vi "senix sonic.vi"() -> ()   [LabVIEW 2014]
uses:
  <vilib>/Instr/_visa.llb/VISA Flush IO Buffer Mask.ctl
  <vilib>/Instr/_visa.llb/VISA Configure Serial Port (Instr).vi
panel:
  out "Waveform Chart":dbl(graph)
  out "Distance, in":dbl
  in  "stop":bool
  out "error out":errorcluster
  out "return count":u32
  out "read buffer":string
  in  "VISA resource name":refnum<visa-resource-name>="COM3"
  # "This vi reads a continuous stream of data from the Senix Sonix sensor TSPC-30S1-232\nThe sensor has been configured to stream continuous data using their software SenixView.\nThe serial port setup values are the default for the Senix sensor."
  # "The value 0000 represent \"no read\""
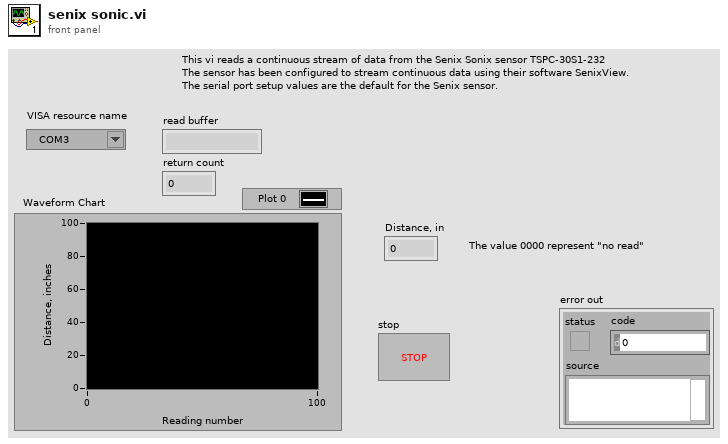
[diagram p1: front panel]
types:
  T1 = typedef "VISA Flush IO Buffer Mask.ctl" = u16
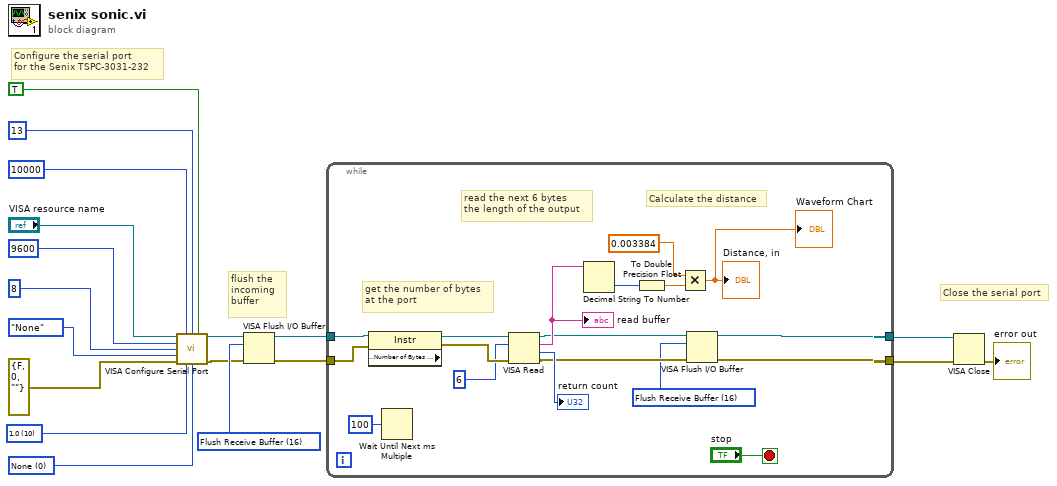
[diagram p0: block diagram]
diagram:
  w5 = T1 16 items=["Flush Receive Buffer"=16, "Write Transmit Buffer to Device"=32, "Flush Receive Buffer (No I/O)"=64, "Flush Transmit Buffer"=128] ("Mask")
  w12 = u16 0 items=["None", "XON/XOFF", "RTS/CTS", "XON/XOFF & RTS/CTS", "DTR/DSR", "XON/XOFF & DTR/DSR"] ("flow control (0:none)")
  w14 = u16 10 items=["1.0"=10, "1.5"=15, "2.0"=20] ("stop bits (10: 1 bit)")
  # "Close the serial port"
  # "flush the \nincoming \nbuffer"
  # "Configure the serial port\nfor the Senix TSPC-3031-232"
  n1 = call-poly "VISA Configure Serial Port"("VISA resource name"="VISA resource name", "timeout (10sec)"=u32 10000, "termination char\n(0xA = '\\n' = LF)"=u8 13 ("termination char\n(0xA = '\\n' = LF)"), "Enable Termination\nChar (T)"=TRUE ("Enable Termination\nChar (T)"), "baud rate (9600)"=u32 9600, "data bits (8)"=u16 8, "parity (0:none)"=enum16{"None", "Odd", "Even", "Mark", "Space"}."None", "error in (no error)"=errorcluster {"status"=FALSE, "code"=0, "source"=""}, "stop bits (10: 1 bit)"=w14, "flow control (0:none)"=w12) -> ("VISA resource name out"=w4:refnum<visa-resource-name>, "error out"=w3:errorcluster)  [unwired: 4 in]
  n2 = VISA Flush I/O Buffer(VISA resource name=w4, mask (16)=w5, error in (no error)=w3) -> (VISA resource name out=w2:refnum<visa-resource-name>, error out=w1:errorcluster)
  n3 = while {
    tunnel: [w25] -> w8
    tunnel: [w24] -> w7
    tunnel: w2 -> [w30]
    tunnel: w1 -> [w29]
    stop <- "stop" stop-if-true
    w21 = T1 16 items=["Flush Receive Buffer"=16, "Write Transmit Buffer to Device"=32, "Flush Receive Buffer (No I/O)"=64, "Flush Transmit Buffer"=128] ("Mask")
    # "Calculate the distance"
    # "read the next 6 bytes\nthe length of the output"
    # "get the number of bytes\nat the port"
    n4 = property class="Instr" props=["Serial Settings:Number of Bytes at Serial Port"](reference=w30, error in=w29) -> (reference out=w36:refnum<visa-resource-name>, error out=w35:errorcluster)  [unwired: 1 out]
    n5 = Wait Until Next ms Multiple(millisecond multiple=u32 100) -> ()  [unwired: 1 out]
    n6 = VISA Read(VISA resource name=w36, byte count=u32 6, error in (no error)=w35) -> (VISA resource name out=w23:refnum<visa-resource-name>, read buffer=w33:string, return count=→"return count":u32, error out=w22:errorcluster)
    "read buffer" <- w33
    n7 = Decimal String To Number(string=w33) -> (number=w28:i32)  [unwired: 2 in, 1 out]
    n8 = To Double Precision Float(number=w28) -> (double precision float=w27:dbl)
    n9 = Multiply(x=0.003384, y=w27) -> (x*y=→"Distance, in" →"Waveform Chart":dbl)
    n10 = VISA Flush I/O Buffer(VISA resource name=w23, mask (16)=w21, error in (no error)=w22) -> (VISA resource name out=w25:refnum<visa-resource-name>, error out=w24:errorcluster)
  }
  n11 = VISA Close(VISA resource name=w8, error in (no error)=w7) -> (error out=→"error out":errorcluster)
